vi "TAT_Com_PLC.vi"() -> ()   [LabVIEW 2017]
uses:
  <vilib>/NI/Modbus Library/API/Wrapper/Create TCP Master.vi
  Global/Global 1.vi
  <vilib>/NI/Modbus Library/API/Master/Modbus Master.lvclass
  <vilib>/NI/Modbus Library/API/Wrapper/API Main.lvlib
panel:
  out "Read From PLC 1":u16[](array[numeric])
  out "Write to PLC":bool[](array[boolean])
  out "error out":errorcluster
  out "Read From PLC":u16[](array[numeric])
  out "PLC STATUS":bool
  in  "error in":errorcluster
  in  "stop":bool
  # "7097 ---D3001"
  # "7108 ---D3012"
  # "Ass & Leak"
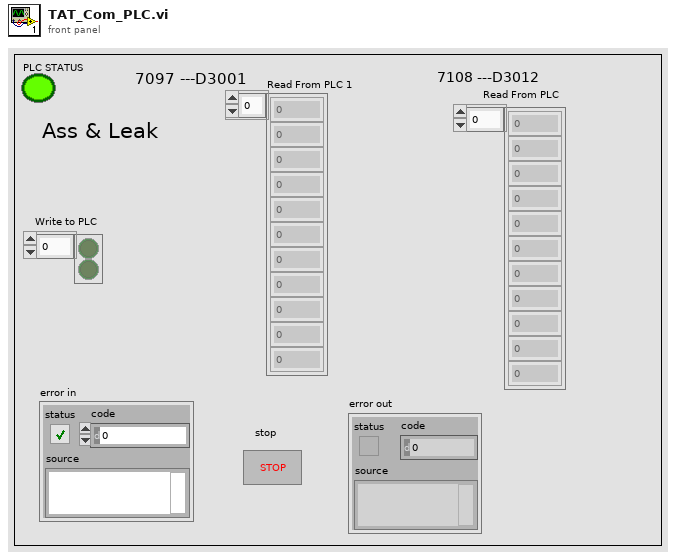
[diagram p1: front panel]
types:
  T1 = enum32{"invalid app kind", "Development System", "Run Time System", "Student Edition", "Embedded LabVIEW", "Evaluation", "Custom"}
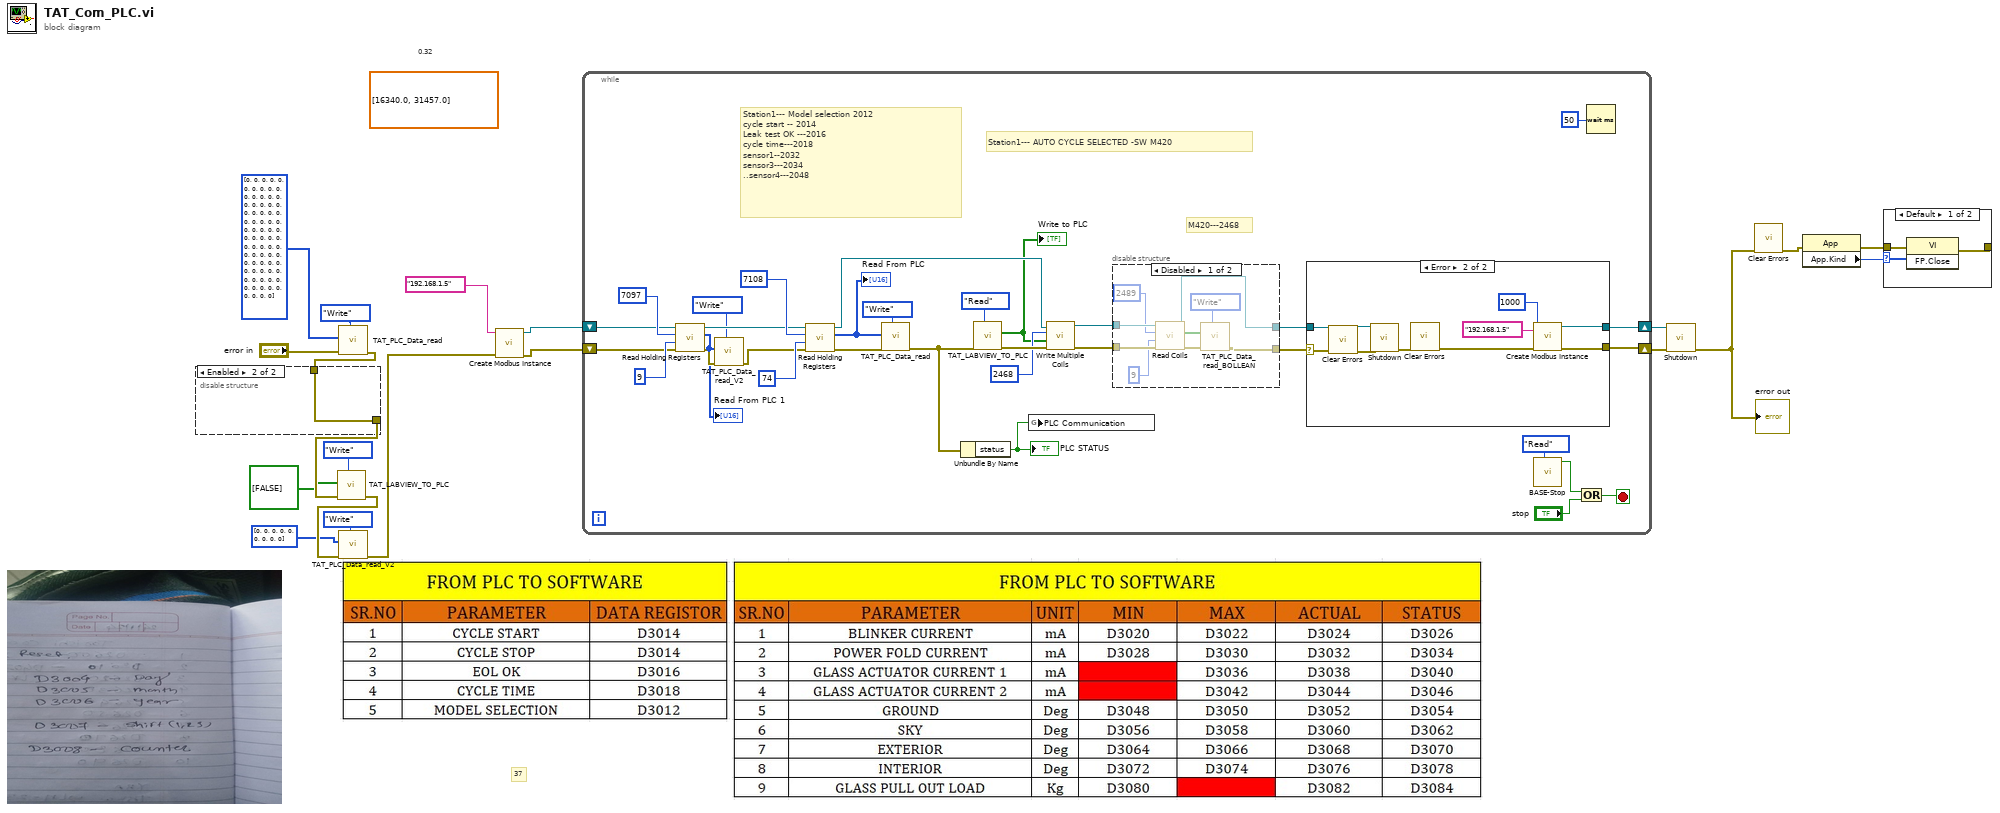
[diagram p0: block diagram]
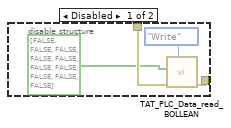
[diagram p2: hidden frame]
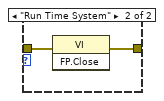
[diagram p5: hidden frame]
diagram:
  (unwired) dbl[] [16340.0, 31457.0] ("register values")
  # "37"
  # "0.32"
  n1 = call "TAT_PLC_Data_read.vi"("Enum"=enum16{"Read", "Write"}."Write", "error in (no error)"="error in", "Array"=u16[] [0, 0, 0, 0, 0, 0, 0, 0, 0, 0, 0, 0, 0, 0, 0, 0, 0, 0, 0, 0, 0, 0, 0, 0, 0, 0, 0, 0, 0, 0, 0, 0, 0, 0, 0, 0, 0, 0, 0, 0, 0, 0, 0, 0, 0, 0, 0, 0, 0, 0, 0, 0, 0, 0, 0, 0, 0, 0, 0, 0, 0, 0, 0, 0, 0, 0, 0, 0, 0, 0, 0, 0, 0, 0] ("Array 3")) -> ("error out"=w10:errorcluster)  [unwired: 7 in, 1 out]
  n2 = disable-structure shown="Enabled" {
    disable-tunnel: w10 -> [w23 w25]
    disable-tunnel: [w21 w25] -> w8
    frame Disabled {
      n3 = call "TAT_PLC_Data_read_BOLLEAN.vi"("Enum"=enum16{"Read", "Write"}."Write", "error in (no error)"=w23, "Array"=bool[] [FALSE, FALSE, FALSE, FALSE, FALSE, FALSE, FALSE, FALSE, FALSE, FALSE]) -> ("error out"=w21:errorcluster)  [unwired: 7 in, 1 out]
    }
    frame Enabled {
    }
  }
  n4 = call "TAT_LABVIEW_TO_PLC.vi"("Enum"=enum16{"Read", "Write"}."Write", "error in (no error)"=w8, "Array"=bool[] [FALSE]) -> ("error out"=w3:errorcluster)  [unwired: 7 in, 1 out]
  n5 = call "TAT_PLC_Data_read_V2.vi"("Enum"=enum16{"Read", "Write"}."Write", "error in (no error)"=w3, "Array"=u16[] [0, 0, 0, 0, 0, 0, 0, 0, 0] ("Array 3")) -> ("error out"=w2:errorcluster)  [unwired: 7 in, 1 out]
  n6 = call-poly <vilib>:"Create Modbus Instance.vi"("error in"=w2, "address"="192.168.1.5") -> ("error out"=w15:errorcluster, "TCP master instance"=w14:refnum<class "Modbus Master.lvclass">)  [unwired: 8 in]
  n7 = while {
    shift-right: [w55] -> w19
    shift-left: w14 -> [w33]
    shift-right: [w54] -> w18
    shift-left: w15 -> [w31]
    stop <- w56 stop-if-true
    # "M420---2468"
    # "Station1--- AUTO CYCLE SELECTED -SW M420"
    # "Station1--- Model selection 2012\ncycle start -- 2014\nLeak test OK ---2016\ncycle time---2018\nsensor1--2032\nsensor3---2034\n..sensor4---2048"
    n8 = call-dynamic "Read Holding Registers.vi"("error in"=w31, "number of inputs"=u16 9, "starting address"=u16 7097, "Modbus master in"=w33) -> ("error out"=w30:errorcluster, "register values"=w28:u16[], "Modbus master out"=w32:refnum<class "Modbus Master.lvclass">)  [unwired: 5 in]
    "Read From PLC 1" <- w28
    n9 = call "TAT_PLC_Data_read_V2.vi"("Enum"=enum16{"Read", "Write"}."Write", "error in (no error)"=w30, "Array"=w28) -> ("error out"=w29:errorcluster)  [unwired: 7 in, 1 out]
    n10 = call-dynamic "Read Holding Registers.vi"("error in"=w29, "number of inputs"=u16 74, "starting address"=u16 7108 ("starting address 2"), "Modbus master in"=w32) -> ("error out"=w49:errorcluster, "register values"=w42:u16[], "Modbus master out"=w48:refnum<class "Modbus Master.lvclass">)  [unwired: 5 in]
    "Read From PLC" <- w42
    n11 = call "TAT_PLC_Data_read.vi"("Enum"=enum16{"Read", "Write"}."Write", "error in (no error)"=w49, "Array"=w42) -> ("error out"=w26:errorcluster)  [unwired: 7 in, 1 out]
    n12 = Unbundle By Name(w26) -> ("status"=w36:bool)
    "PLC STATUS" <- w36
    n13 = call "TAT_LABVIEW_TO_PLC.vi"("Enum"=enum16{"Read", "Write"}."Read", "error in (no error)"=w26) -> ("error out"=w46:errorcluster, "Array 2"=w41:bool[])  [unwired: 8 in]
    "Write to PLC" <- w41
    n14 = global write "Global 1.vi" "PLC Communication"(w36) -> ()
    n15 = call-dynamic "Write Multiple Coils.vi"("error in"=w46, "coils to write"=w41, "starting address"=u16 2468, "Modbus master in"=w48) -> ("error out"=w40:errorcluster, "Modbus master out"=w39:refnum<class "Modbus Master.lvclass">)  [unwired: 6 in]
    n16 = disable-structure shown="Disabled" {
      disable-tunnel: w40 -> [w65 w67]
      disable-tunnel: w39 -> [w64 w68]
      disable-tunnel: [w63 w68] -> w38
      disable-tunnel: [w58 w67] -> w37
      frame Disabled {
        n17 = call-dynamic "Read Coils.vi"("error in"=w65, "number of inputs"=u16 9, "starting address"=u16 2489, "Modbus master in"=w64) -> ("error out"=w59:errorcluster, "coils"=w60:bool[], "Modbus master out"=w63:refnum<class "Modbus Master.lvclass">)  [unwired: 5 in]
        n18 = call "TAT_PLC_Data_read_BOLLEAN.vi"("Enum"=enum16{"Read", "Write"}."Write", "error in (no error)"=w59, "Array"=w60) -> ("error out"=w58:errorcluster)  [unwired: 7 in, 1 out]
      }
      frame Enabled {
      }
    }
    n19 = case shown="Error" w37 {
      selector: w37 -> [w69 w79]
      tunnel: w38 -> [w70 w77]
      tunnel: [w70 w73] -> w55
      tunnel: [w69 w72] -> w54
      frame No Error {
      }
      frame Error {
        n20 = call <vilib>:"Clear Errors.vi"("error in (no error)"=w79) -> ("error out"=w78:errorcluster)  [unwired: 5 in, 1 out]
        n21 = call-dynamic "Shutdown.vi"("error in"=w78, "Modbus master in"=w77) -> ("error out"=w76:errorcluster)  [unwired: 9 in]
        n22 = call <vilib>:"Clear Errors.vi"("error in (no error)"=w76) -> ("error out"=w74:errorcluster)  [unwired: 5 in, 1 out]
        n23 = call-poly <vilib>:"Create Modbus Instance.vi"("error in"=w74, "connect timeout ms"=1000, "address"="192.168.1.5") -> ("error out"=w72:errorcluster, "TCP master instance"=w73:refnum<class "Modbus Master.lvclass">)  [unwired: 7 in]
      }
    }
    n24 = call "BASE-Stop.vi"("Enum"=enum16{"Read", "Write"}."Read") -> ("Stop"=w43:bool)  [unwired: 10 in]
    n25 = Or(x=w43, y="stop") -> (x .or. y?=w56:bool)
    n26 = Wait (ms)(milliseconds to wait=u32 50) -> ()  [unwired: 1 out]
  }
  n27 = call-dynamic "Shutdown.vi"("error in"=w18, "Modbus master in"=w19) -> ("error out"=w6:errorcluster)  [unwired: 9 in]
  "error out" <- w6
  n28 = call <vilib>:"Clear Errors.vi"("error in (no error)"=w6) -> ("error out"=w5:errorcluster)  [unwired: 5 in, 1 out]
  n29 = property class="App"(error in=w5) -> (error out=w16:errorcluster, "App.Kind"=w17:T1)  [unwired: 1 in, 1 out]
  n30 = case shown="Default" w17 {
    tunnel: w16 -> [w81 w83]
    tunnel: [w80 w82] -> _
    frame Default {
      n31 = invoke class="VI" method="FP.Close"(error in=w81) -> (error out=w80:errorcluster)  [unwired: 2 in, 2 out]
    }
    frame "Run Time System" {
      n32 = invoke class="VI" method="FP.Close"(error in=w83) -> (error out=w82:errorcluster)  [unwired: 2 in, 2 out]
    }
  }
